vi "Main - Independent.vi"() -> ()   [LabVIEW 2013]
panel:
  in  "Output Dir":path=path "D:/Development/Projects/LQWidgets/src/LabVIEW"
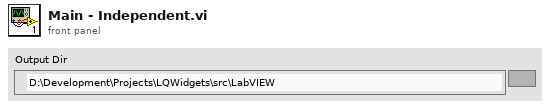
[diagram p1: front panel]
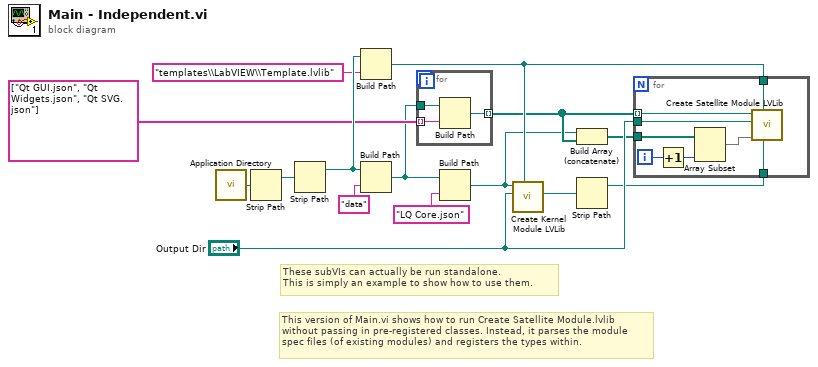
[diagram p0: block diagram]
diagram:
  # "This version of Main.vi shows how to run Create Satellite Module.lvlib\nwithout passing in pre-registered classes. Instead, it parses the module\nspec files (of existing modules) and registers the types within."
  # "These subVIs can actually be run standalone.\nThis is simply an example to show how to use them."
  n1 = call <vilib>:"Application Directory.vi"() -> ("Application Directory"=w15:path)
  n2 = Strip Path(path=w15) -> (stripped path=w13:path)  [unwired: 1 out]
  n3 = Strip Path(path=w13) -> (stripped path=w10:path)  [unwired: 1 out]
  n4 = Build Path(base path=w10, name or relative path="templates\\LabVIEW\\Template.lvlib") -> (appended path=w8:path)
  n5 = Build Path(base path=w10, name or relative path="data") -> (appended path=w6:path)
  n6 = for {
    tunnel: string[] ["Qt GUI.json", "Qt Widgets.json", "Qt SVG.json"] -> [w18] mode=indexing
    tunnel: w6 -> [w17]
    tunnel: [w16] -> w4 mode=indexing
    n7 = Build Path(base path=w17, name or relative path=w18) -> (appended path=w16:path)
  }
  n8 = Build Path(base path=w6, name or relative path="LQ Core.json") -> (appended path=w1:path)
  n9 = call "Create Kernel Module LVLib.vi"("Template LVLib Path"=w8, "Output Dir"="Output Dir", "Module Spec. File"=w1) -> ("Module LVLib Path"=w2:path)  [unwired: 7 in, 1 out]
  n10 = Build Array (concatenate)(w1, w4) -> (w3:path[])
  n11 = Strip Path(path=w2) -> (stripped path=w5:path)  [unwired: 1 out]
  n12 = for {
    tunnel: "Output Dir" -> [w26]
    tunnel: w4 -> [w25] mode=indexing
    tunnel: w8 -> [w24]
    tunnel: w5 -> [w23]
    tunnel: w3 -> [w22]
    i -> [w21]
    n13 = Increment(x=w21) -> (x+1=w19:i32)
    n14 = Array Subset(array=w22, length=w19) -> (w20:path[])  [unwired: 1 in]
    n15 = call "Create Satellite Module LVLib.vi"("Kernel LVLib Dir"=w23, "Template LVLib Path"=w24, "Dependency Spec Files"=w20, "Output Dir"=w26, "Module Spec. File"=w25) -> ()  [unwired: 5 in, 2 out]
  }
